vi "SetState.vi"(8 "error in (no error)":errorcluster, 10 "State":T1, 11 "DriveBase in":refnum<class "DriveBase.lvclass">) -> (0 "error out":errorcluster, 3 "DriveBase out":refnum<class "DriveBase.lvclass">)   [LabVIEW 2016, in "DriveBase.lvclass"]
uses:
  DriveBase.lvclass
  DriveStates.ctl
  DriveBase.lvclass/DriveBase.ctl
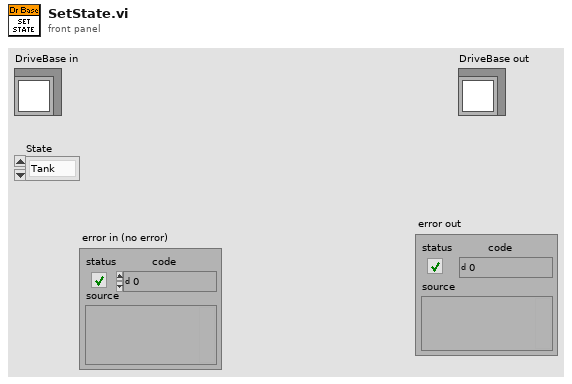
[diagram p1: front panel]
types:
  T1 = typedef "DriveBase.lvclass/DriveStates.ctl" = enum16{"Tank", "Arcade", "DriveStraight"}
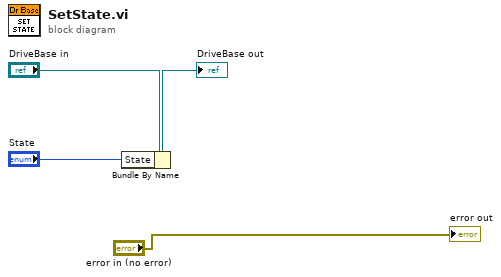
[diagram p0: block diagram]
diagram:
  n1 = Bundle By Name(cluster="DriveBase in", "State"="State") -> (→"DriveBase out":refnum<class "DriveBase.lvclass">)
  "error out" <- "error in (no error)"
